vi "Unregister Callbacks.vi"(8 "error in (no error)":errorcluster, 11 "Callback":T1) -> (0 "error out":errorcluster)   [LabVIEW 2020, in "NI_VS UI Single Node Browser.lvlib"]
uses:
  <vilib>/NI VeriStand/UI Controls/Single Node Browser/NI_VS UI Single Node Browser.lvlib
  <vilib>/NI VeriStand/UI Controls/Single Node Browser/Callback Type.ctl
  <vilib>/NI VeriStand/UI Controls/Single Node Browser/Net Event Data.ctl
  <vilib>/NI VeriStand/UI Controls/Single Node Browser/Net Event.ctl
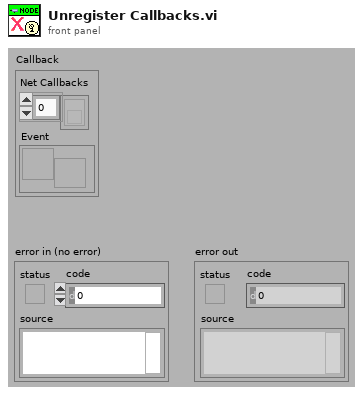
[diagram p1: front panel]
types:
  T1 = typedef "NI_VS UI Single Node Browser.lvlib/Callback Type.ctl" = cluster{"Net Callbacks":refnum<k27>[], "Event":refnum<user-event>}
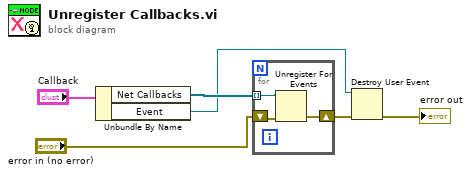
[diagram p0: block diagram]
diagram:
  n1 = Unbundle By Name("Callback") -> ("Net Callbacks"=w5:refnum<k27>[], "Event"=w4:refnum<user-event>)
  n2 = for {
    tunnel: w5 -> [w9] mode=indexing
    shift-right: [w7] -> w3
    shift-left: "error in (no error)" -> [w8]
    n3 = Unregister For Events(event registration refnum=w9, error in=w8) -> (error out=w7:errorcluster)
  }
  n4 = Destroy User Event(user event=w4, error in=w3) -> (error out=→"error out":errorcluster)
